vi "MP_LaunchMatlabScript3.vi"(8 "error in (no error)":errorcluster, 11 "matlab script with path":path) -> (0 "error out":errorcluster, 2 "standard error":string, 3 "standard output":string, 4 "OS Name":string, 5 "computed command line":string)   [LabVIEW 2022 SP3]
doc: "Launch matlab with the script passed as parameter. \nThe script and the VI MUST be in the same directory!\n\nWorks on OSX, Windows and Linux On Linux, assume Ubuntu (salles CO) and current 2013 \"matlab\" CMD. \nOn OSX, search for the latest release of matlab, see diagram.\nOn Windows, assume \"matlab\" command exists.\n\nThere is demo script if needed, see the diagram to activate it.\n\nChS. 2013-21, updated to use '-batch' instead of '-r'"
uses:
  <vilib>/Utility/sysdir.llb/System Directory Type.ctl
panel:
  out "is shortcut":bool
  out "is directory":bool
  # "Since ML 2018 use \"-batch\""
  # "Added script path"
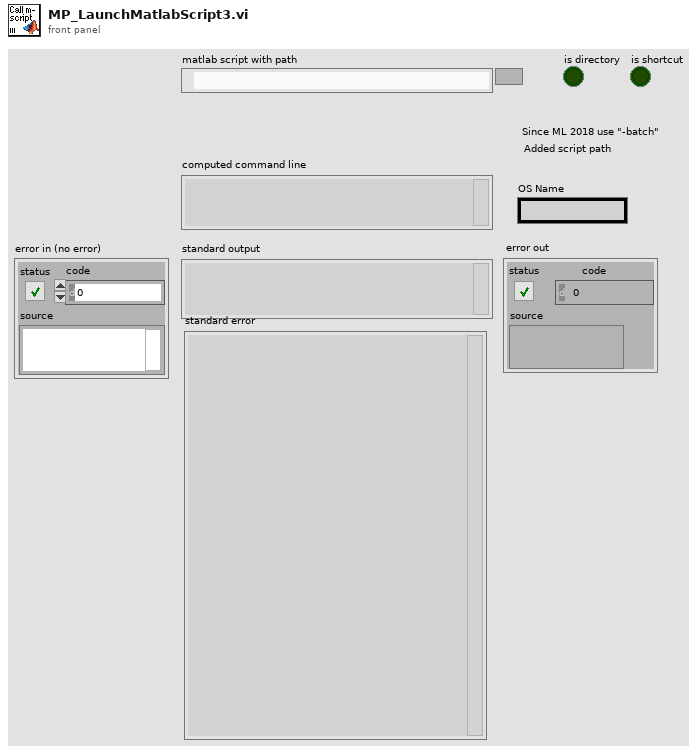
[diagram p1: front panel]
types:
  T1 = enum16{"open", "replace", "create", "open or create", "replace or create", "replace or create with confirmation"}
  T2 = typedef "System Directory Type.ctl" = i32
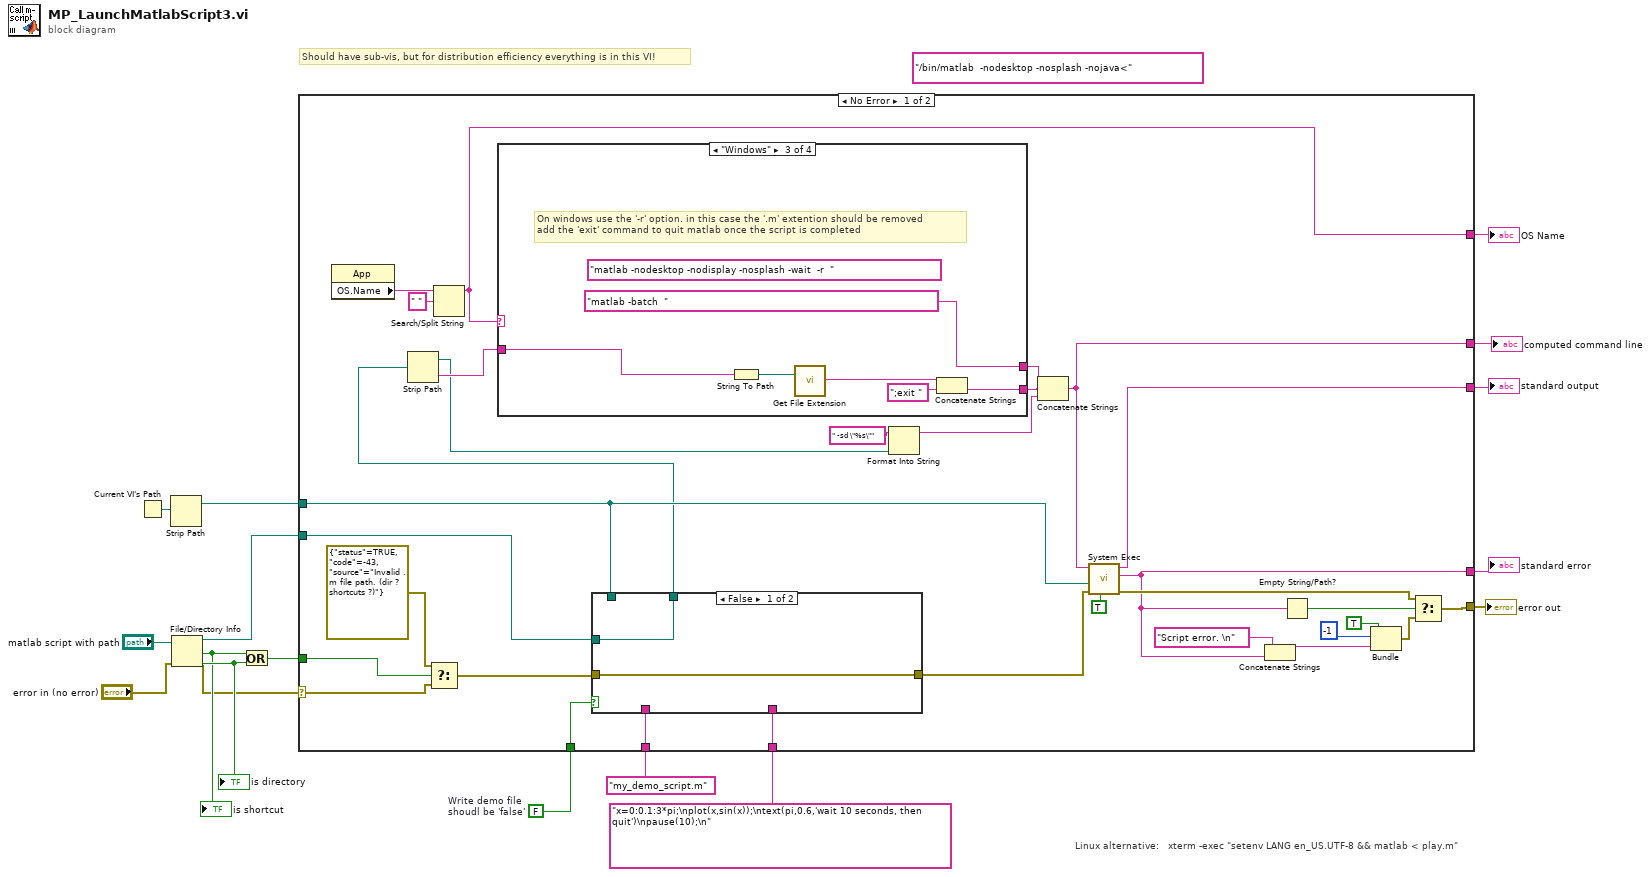
[diagram p0: block diagram]
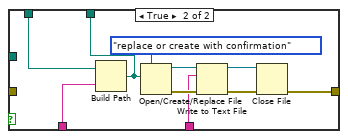
[diagram p2: hidden frame]
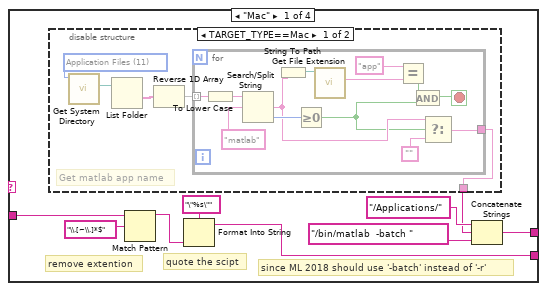
[diagram p3: hidden frame]
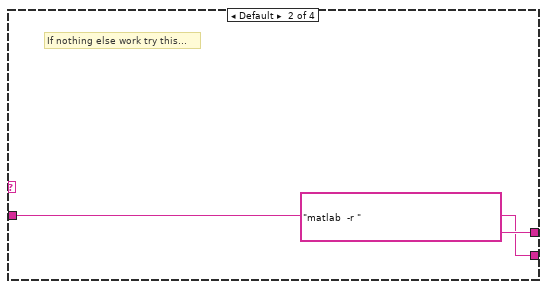
[diagram p5: hidden frame]
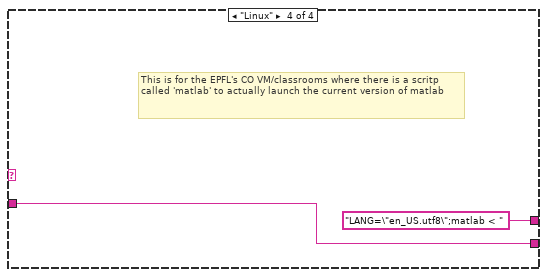
[diagram p6: hidden frame]
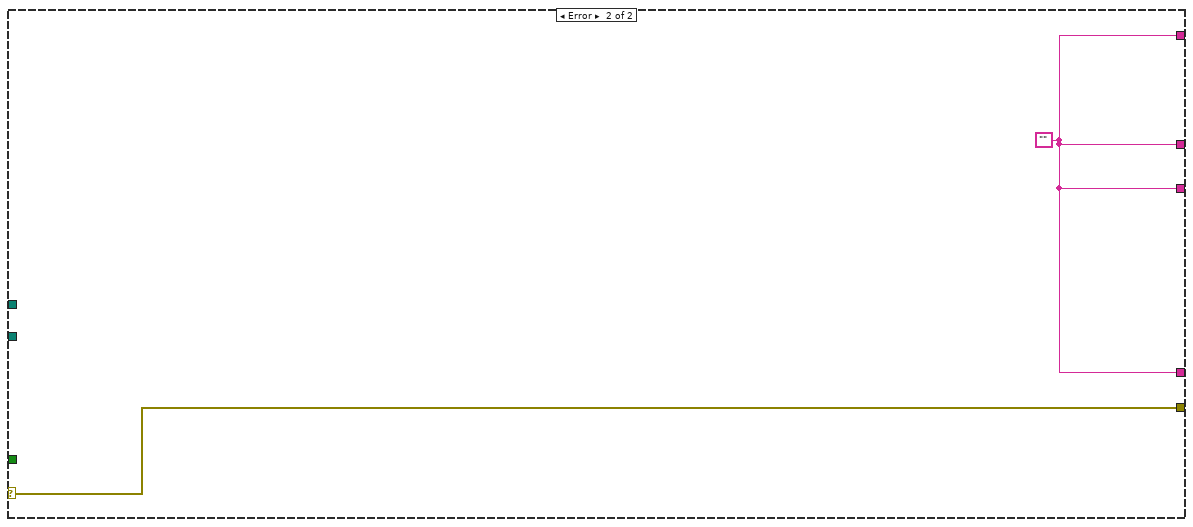
[diagram p7: hidden frame]
diagram:
  (unwired) "/bin/matlab  -nodesktop -nosplash -nojava<" ("name or relative path")
  w10 = FALSE  # Write demo file shoudl be 'false'
  # "Should have sub-vis, but for distribution efficiency everything is in this VI!"
  # "Linux alternative:   xterm -exec \"setenv LANG en_US.UTF-8 && matlab < play.m\""
  n1 = Current VI's Path() -> (path=w9:path)
  n2 = Strip Path(path=w9) -> (stripped path=w8:path)  [unwired: 1 out]
  n3 = File/Directory Info(path="matlab script with path", error in="error in (no error)") -> (path out=w6:path, directory=w5:bool, error out=w1:errorcluster, shortcut=w4:bool)  [unwired: 3 out]
  "is directory" <- w5
  "is shortcut" <- w4
  n4 = Or(x=w4, y=w5) -> (x .or. y?=w3:bool)
  n5 = case shown="No Error" w1 {
    selector: w1 -> [w48 w100]
    tunnel: [w49 w99] -> w17
    tunnel: [w39 w99] -> w16
    tunnel: [w41 w100] -> w15
    tunnel: [w44 w99] -> w14
    tunnel: [w32 w99] -> w13
    tunnel: "x=0:0.1:3*pi;\nplot(x,sin(x));\ntext(pi,0.6,'wait 10 seconds, then quit')\npause(10);\n" ("text") -> [w30 _]
    tunnel: "my_demo_script.m" ("name or relative path") -> [w29 _]
    tunnel: w10 -> [w28 _]
    tunnel: w8 -> [w26 _]
    tunnel: w6 -> [w19 _]
    tunnel: w3 -> [w21 _]
    frame No Error {
      n6 = property class="App"() -> ("OS.Name"=w33:string)  [unwired: 2 in, 2 out]
      n7 = Select(t=errorcluster {"status"=TRUE, "code"=-43, "source"="Invalid .m file path. (dir ? shortcuts ?)"} ("error constant"), s=w21, f=w48) -> (s? t:f=w46:errorcluster)
      n8 = Search/Split String(string=w33, search string/char (-)=" ") -> (substring before match=w32:string)  [unwired: 1 in, 2 out]
      n9 = case shown="False" w28 {
        tunnel: [w51 w57] -> w20
        tunnel: w26 -> [_ w55]
        tunnel: w46 -> [w51 _]
        tunnel: w30 -> [_ w54]
        tunnel: w29 -> [_ w53]
        tunnel: [w50 w52] -> w18
        tunnel: w19 -> [w50 _]
        frame False {
        }
        frame True {
          n10 = Build Path(base path=w55, name or relative path=w53) -> (appended path=w52:path)
          n11 = Open/Create/Replace File(file path (use dialog)=w52, operation (0:open)=T1."replace or create with confirmation") -> (refnum out=w58:refnum<file>, error out=w61:errorcluster)  [unwired: 4 in, 1 out]
          n12 = Write to Text File(file (use dialog)=w58, text=w54, error in=w61) -> (refnum out=w59:refnum<file>, error out=w60:errorcluster)  [unwired: 1 in, 1 out]
          n13 = Close File(refnum=w59, error in=w60) -> (error out=w57:errorcluster)  [unwired: 1 out]
        }
      }
      n14 = Strip Path(path=w18) -> (stripped path=w23:path, name=w25:string)
      n15 = case shown="\"Windows\"" w32 {
        tunnel: [w68 "matlab  -r " ("name or relative path") "matlab -batch  " ("name or relative path") "LANG=\"en_US.utf8\";matlab < "] -> w45
        tunnel: w25 -> [w65 w89 w95 w97]
        tunnel: [w63 w89 w92 w97] -> w34
        frame "Mac" {
          # "since ML 2018 should use '-batch' instead of '-r'"
          # "quote the scipt"
          # "remove extention"
          n16 = disable-structure shown="TARGET_TYPE==Mac" {
            disable-tunnel: [w71 _] -> w67
            frame condition #0 {
              w75 = T2 11 items=["User Home"=0, "User Desktop"=1, "User Documents"=2, "User Application Data"=3, "User Preferences"=4, "User Temporary"=5, "Public Documents"=6, "Public Application Data"=7, "Public Preferences"=8, "Public Cache"=13, "System Core Libraries"=9, "System Installed Libraries"=10, "Application Files"=11, "Boot Volume Root"=12] ("system directory type")
              # "Get matlab app name"
              n17 = call <vilib>:"Get System Directory.vi"("system directory type"=w75) -> ("system directory"=w72:path)  [unwired: 10 in]
              n18 = List Folder(path=w72) -> (folder names=w74:string[])  [unwired: 3 in, 3 out]
              n19 = Reverse 1D Array(array=w74) -> (reversed array=w73:string[])
              n20 = for {
                tunnel: w73 -> [w88] mode=indexing
                tunnel: [w79] -> w71
                stop <- w81 stop-if-true
                n21 = To Lower Case(string=w88) -> (all lower case string=w87:string)
                n22 = Search/Split String(string=w87, search string/char (-)="matlab") -> (match + rest of string=w78:string, offset of match=w85:i32)  [unwired: 1 in, 1 out]
                n23 = String To Path(string=w78) -> (path=w84:path)
                n24 = Greater Or Equal To 0?(x=w85) -> (x >= 0?=w77:bool)
                n25 = call <vilib>:"Get File Extension.vi"("file"=w84) -> ("lowercase file extension"=w82:string)  [unwired: 6 in, 4 out]
                n26 = Equal?(x="app", y=w82) -> (x = y?=w80:bool)
                n27 = And(x=w80, y=w77) -> (x .and. y?=w81:bool)
                n28 = Select(t=w78, s=w77, f="") -> (s? t:f=w79:string)
              }
            }
            frame condition #1 (active) {
            }
          }
          n29 = Match Pattern(string=w65, regular expression="\\.[~\\.]*$") -> (before substring=w64:string)  [unwired: 1 in, 3 out]
          n30 = Format Into String(format string="\"%s\"", w64) -> (resulting string=w63:string)  [unwired: 2 in, 1 out]
          n31 = Concatenate Strings("/Applications/" ("name or relative path"), w67, "/bin/matlab  -batch " ("name or relative path")) -> (w68:string)
        }
        frame Default {
          # "If nothing else work try this..."
        }
        frame "Windows" {
          (unwired) "matlab -nodesktop -nodisplay -nosplash -wait  -r  " ("name or relative path")
          # "On windows use the '-r' option. in this case the '.m' extention should be removed\nadd the 'exit' command to quit matlab once the script is completed"
          n32 = String To Path(string=w95) -> (path=w94:path)
          n33 = call <vilib>:"Get File Extension.vi"("file"=w94) -> ("filename without extension"=w93:string)  [unwired: 6 in, 4 out]
          n34 = Concatenate Strings(w93, ";exit " ("string")) -> (w92:string)
        }
        frame "Linux" {
          # "This is for the EPFL's CO VM/classrooms where there is a scritp called 'matlab' to actually launch the current version of matlab"
        }
      }
      n35 = Format Into String(format string=" -sd \"%s\"", w23) -> (resulting string=w24:string)  [unwired: 2 in, 1 out]
      n36 = Concatenate Strings(w45, w34, w24) -> (w44:string)
      n37 = call <vilib>:"System Exec.vi"("run minimized? (F)"=TRUE, "error in (no error)"=w20, "working directory"=w26, "command line"=w44) -> ("error out"=w42:errorcluster, "standard error"=w39:string, "standard output"=w49:string)  [unwired: 4 in, 1 out]
      n38 = Concatenate Strings("Script error. \n" ("source"), w39) -> (w36:string)
      n39 = Empty String/Path?(string/path=w39) -> (empty?=w43:bool)
      n40 = Bundle("status"=TRUE, "code"=-1, w36) -> (w40:cluster{"status":bool, "code":i32, string})  [unwired: 1 in]
      n41 = Select(t=w42, s=w43, f=w40) -> (s? t:f=w41:errorcluster)
    }
    frame Error {
      w99 = "" ("standard error")
    }
  }
  "standard output" <- w17
  "standard error" <- w16
  "error out" <- w15
  "computed command line" <- w14
  "OS Name" <- w13
